vi "Initialise Laser.vi"(5 "Endpoint":refnum<class "Vector 2D.lvclass">, 7 "Origin":refnum<class "Vector 2D.lvclass">, 9 "Colour":u32(colorbox), 10 "Damage":i32=100, 11 "Player":T1) -> (3 "Laser out":refnum<class "Laser.lvclass">)   [LabVIEW 2021, in "Laser.lvclass"]
uses:
  Laser.lvclass
  Vector 2D/Vector 2D.lvclass
  Laser.lvclass/Laser.ctl
  Weapon/Weapon.lvclass
  Actors/Main Controller/Actor/Player.ctl
  Actors/Main Controller/Actor/Main Controller Actor.lvclass
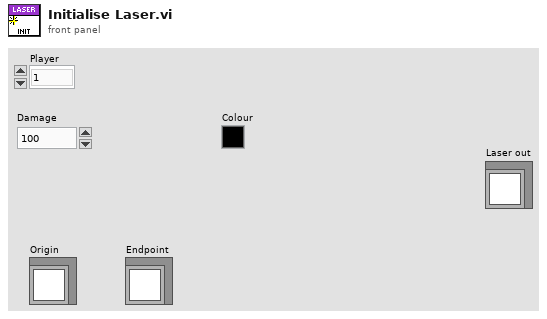
[diagram p1: front panel]
types:
  T1 = typedef "Main Controller Actor.lvclass/Player.ctl" = enum16{"1", "2"}
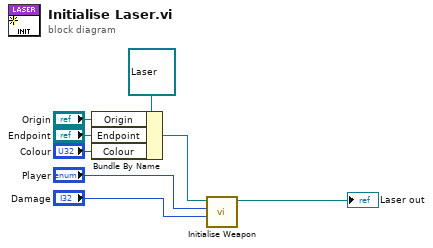
[diagram p0: block diagram]
diagram:
  n1 = Bundle By Name(cluster=refnum<class "Laser.lvclass"> refnum ("Ship"), "Origin"="Origin", "Endpoint"="Endpoint", "Colour"="Colour") -> (w4:refnum<class "Laser.lvclass">)
  n2 = call "Initialise Weapon.vi"("Damage"="Damage", "Player"="Player", "Weapon in"=w4) -> ("Weapon out"=→"Laser out":refnum<class "Laser.lvclass">)  [unwired: 8 in]
